vi "Is Doors Locked.vi"(8 "error in":errorcluster) -> (0 "error out":errorcluster, 1 "Rear Doors Closed":bool, 2 "Front Right Door Closed":bool, 3 "Front Left Doors Closed":bool, 4 "Doors Locked":bool)   [LabVIEW 2010]
doc: "This function verifies all test set doors are closed and locked. If any of the doors are open or unlocked, then an error is returned."
uses:
  <vilib>/DAQmx/read.llb/DAQmx Read (Digital U8 1Chan 1Samp).vi
  <vilib>/DAQmx/create/channels.llb/DAQmx Create Channel (DI-Digital Input).vi
  <vilib>/daqmx/miscellaneous.llb/DAQmx Fill In Error Info.vi
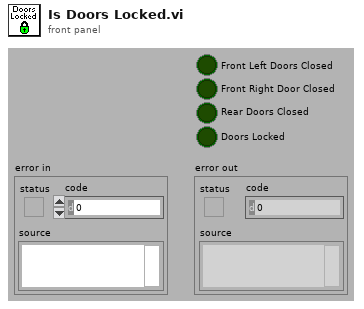
[diagram p1: front panel]
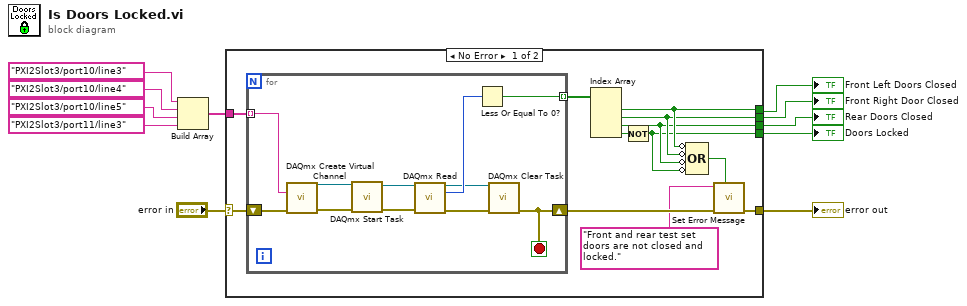
[diagram p0: block diagram]
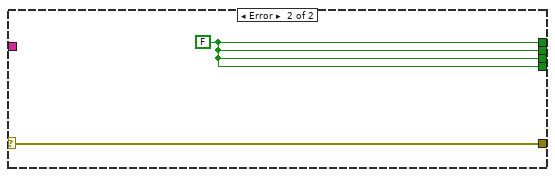
[diagram p2: hidden frame]
diagram:
  n1 = Build Array(tag "PXI2Slot3/port10/line3" ("Lines"), tag "PXI2Slot3/port10/line4" ("Lines"), tag "PXI2Slot3/port10/line5" ("Lines"), tag "PXI2Slot3/port11/line3" ("Lines")) -> (w10:tag[])
  n2 = case shown="No Error" "error in" {
    selector: "error in" -> [w22 w36]
    tunnel: w10 -> [w23 _]
    tunnel: [w18 w36] -> w8
    tunnel: [w16 w35] -> w7
    tunnel: [w15 w35] -> w4
    tunnel: [w13 w35] -> w6
    tunnel: [w14 w35] -> w5
    frame No Error {
      n3 = for {
        shift-right: [w24] -> w19
        shift-left: w22 -> [w27]
        tunnel: [w26] -> w21 mode=indexing
        tunnel: w23 -> [w25] mode=indexing
        stop <- w24 stop-if-true
        n4 = call-poly <vilib>:"DAQmx Create Virtual Channel.vi"("lines"=w25, "error in"=w27) -> ("task out"=w34:refnum<k21>, "error out"=w33:errorcluster)  [unwired: 12 in]
        n5 = call <vilib>:"DAQmx Start Task.vi"("task/channels in"=w34, "error in"=w33) -> ("task out"=w31:refnum<k21>, "error out"=w32:errorcluster)  [unwired: 12 in]
        n6 = call-poly <vilib>:"DAQmx Read.vi"("task/channels in"=w31, "error in"=w32) -> ("task out"=w29:refnum<k21>, "data"=w30:u8, "error out"=w28:errorcluster)  [unwired: 11 in]
        n7 = Less Or Equal To 0?(x=w30) -> (x <= 0?=w26:bool)
        n8 = call <vilib>:"DAQmx Clear Task.vi"("task in"=w29, "error in"=w28) -> ("error out"=w24:errorcluster)  [unwired: 13 in]
      }
      n9 = Index Array(array=w21) -> (element #1=w16:bool, element #2=w15:bool, element #3=w14:bool, element #4=w20:bool)  [unwired: 4 in]
      n10 = Not(x=w20) -> (.not. x?=w13:bool)
      n11 = Compound Arithmetic op=OR(invert w16, invert w15, invert w14, invert w13) -> (w17:bool)
      n12 = call "Set Error Message.vi"("Enable (T)"=w17, "error in"=w19, "Message"="Front and rear test set doors are not closed and locked.") -> ("error out"=w18:errorcluster)  [unwired: 5 in]
    }
    frame Error {
      w35 = FALSE
    }
  }
  "Doors Locked" <- w6
  "Rear Doors Closed" <- w5
  "Front Right Door Closed" <- w4
  "Front Left Doors Closed" <- w7
  "error out" <- w8
